vi "get_notebook.vi"(8 "error in (no error)":errorcluster, 11 "GenericComponent in":refnum<class "GenericComponent.lvclass">) -> (0 "error out":errorcluster, 2 "notebook":refnum<class "Notebook.lvclass">, 3 "GenericComponent out":refnum<class "GenericComponent.lvclass">)   [LabVIEW 2010, in "GenericComponent.lvclass"]
uses:
  GenericComponent.lvclass
  NoteBook/Notebook/Notebook.lvclass
  class_data.vi
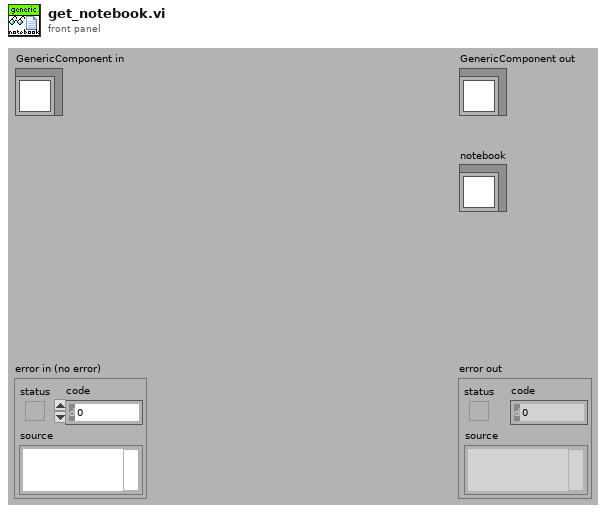
[diagram p1: front panel]
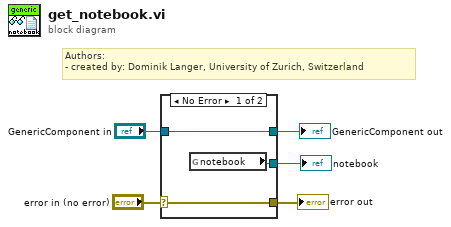
[diagram p0: block diagram]
diagram:
  # "Authors: \n- created by: Dominik Langer, University of Zurich, Switzerland"
  n1 = case shown="No Error" "error in (no error)" {
    selector: "error in (no error)" -> [w7 w10]
    tunnel: [w7 w10] -> w4
    tunnel: [w8 w9] -> w2
    tunnel: "GenericComponent in" -> [w8 w9]
    tunnel: [w6 _] -> w1
    frame No Error {
      n2 = global read "class_data.vi" "notebook"() -> (w6:refnum<class "Notebook.lvclass">)
    }
    frame Error {
    }
  }
  "error out" <- w4
  "GenericComponent out" <- w2
  "notebook" <- w1
